vi "Instrument.Write Configuration File.vi"(8 "error in (no error)":errorcluster, 11 "Instrument in":refnum<class "Instrument.lvclass">) -> (0 "error out":errorcluster, 3 "Instrument out":refnum<class "Instrument.lvclass">)   [LabVIEW 2016, in "Instrument.lvclass"]
uses:
  Instrument.lvclass
  Instrument.lvclass/Instrument.ctl
  Configuration/Configuration.lvclass
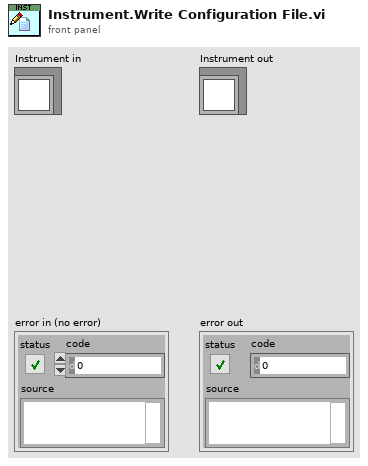
[diagram p1: front panel]
types:
  T1 = typedef "Instrument.lvclass/Configuration--Cluster.ctl" = cluster{"Hardware":T2, "SMO":T3, "DSC":T5}
  T2 = typedef "Instrument.lvclass/HW Configuration--Cluster.ctl" = cluster{"Address":string, "Type":string, "COM Type":string}
  T3 = typedef "Instrument.lvclass/SMO Configuration--Cluster.ctl" = cluster{"Address":string, "Port":u16, "RC Type":T4}
  T4 = typedef "Instrument.lvclass/SMO RC Type--enum.ctl" = enum16{"RC", "STM", "ZMQ"}
  T5 = typedef "Instrument.lvclass/DSC Configuration--Cluster.ctl" = cluster{"Process Name":string}
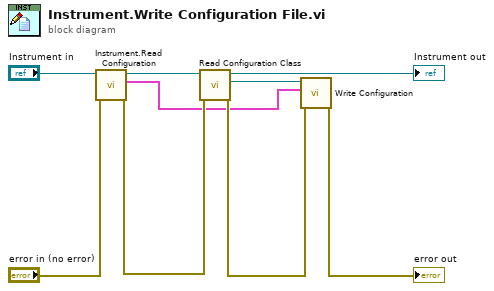
[diagram p0: block diagram]
diagram:
  n1 = call "Instrument.Read Configuration.vi"("error in (no error)"="error in (no error)", "Instrument in"="Instrument in") -> ("error out"=w4:errorcluster, "Instrument Configuration"=w1:T1, "Instrument out"=w2:refnum<class "Instrument.lvclass">)  [unwired: 7 in]
  n2 = call "Read Configuration Class.vi"("error in (no error)"=w4, "Instrument in"=w2) -> ("error out"=w7:errorcluster, "Configuration.lvclass"=w8:refnum<class "Configuration.lvclass">, "Instrument out"=→"Instrument out":refnum<class "Instrument.lvclass">)  [unwired: 7 in]
  n3 = call "Write Configuration.vi"("error in (no error)"=w7, "Variant"=w1, "Configuration in"=w8) -> ("error out"=→"error out":errorcluster)  [unwired: 7 in, 1 out]
